vi "LS370 Change Excitation text in.vi"(0 "command text in":string[](array[string])) -> (1 "Channel":i32=1 min=1 max=16 step=1, 2 "VISA Refnum in":refnum<visa-resource-name>, 3 "Sweep Time (sec)":dbl=3600.0, 4 "extra wait":i32, 5 "Current":u16, 6 "Mode":enum32{"Voltage", "Current"}(ring), 7 "Resistance Range":T1)   [LabVIEW 2024]
uses:
  LS370 Resistance Range.ctl
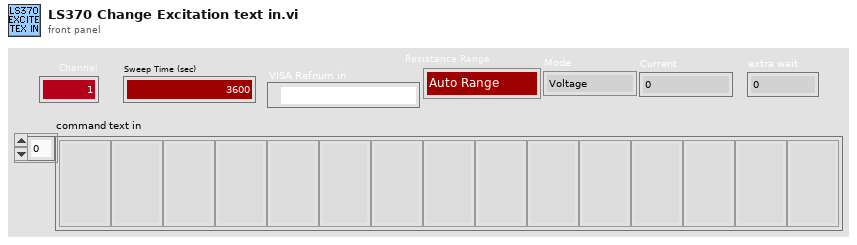
[diagram p1: front panel]
types:
  T1 = typedef "LS370 Resistance Range.ctl" = enum16{"Auto Range", "2.00 mΩ", "6.32 mΩ", "20.0 mΩ", "63.2 mΩ", "200 mΩ", "632 mΩ", "2.00 Ω", "6.32 Ω", "20.0 Ω", "63.2 Ω", "200 Ω", "632 Ω", "2.00 kΩ", "6.32 kΩ", "20.0 kΩ", "63.2 kΩ", "200 kΩ", "632 kΩ", "2.00 MΩ", "6.32 MΩ", "20.0 MΩ", "63.2 MΩ"}
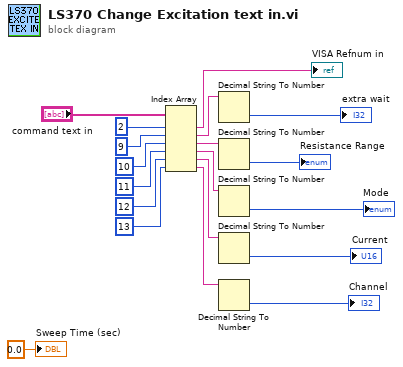
[diagram p0: block diagram]
diagram:
  n1 = Index Array(array="command text in", index #1=2 ("index"), index #2=9 ("index"), index #3=10 ("index"), index #4=11 ("index"), index #5=12 ("index"), index #6=13 ("index")) -> (element #1=→"VISA Refnum in":string, element #2=w16:string, element #3=w3:string, element #4=w2:string, element #5=w1:string, element #6=w8:string)
  n2 = Decimal String To Number(string=w16) -> (number=→"extra wait":i32)  [unwired: 2 in, 1 out]
  n3 = Decimal String To Number(string=w3) -> (number=→"Resistance Range":i32)  [unwired: 2 in, 1 out]
  n4 = Decimal String To Number(string=w2) -> (number=→"Mode":i32)  [unwired: 2 in, 1 out]
  n5 = Decimal String To Number(string=w1) -> (number=→"Current":i32)  [unwired: 2 in, 1 out]
  n6 = Decimal String To Number(string=w8) -> (number=→"Channel":i32)  [unwired: 2 in, 1 out]
  "Sweep Time (sec)" <- 0.0 ("Sweep Time (sec)")
